vi "WSVCAP SHL Host TL RFFE Write - Multiple DUTs - Common Data.vi"(0 "Data Out":string, 11 "error in":errorcluster, 12 "FPGA":T1, 13 "DUT Mask (All)":bool[](array[boolean])=[TRUE, TRUE, TRUE, TRUE, TRUE, TRUE, TRUE, TRUE, TRUE, TRUE, TRUE, TRUE, TRUE, TRUE, TRUE, TRUE, TRUE, TRUE, TRUE, TRUE, TRUE, TRUE, TRUE, TRUE, TRUE, TRUE, TRUE, TRUE, TRUE, TRUE, TRUE, TRUE, TRUE, TRUE, TRUE, TRUE], 14 "Log (T)":bool=TRUE) -> (15 "error out":errorcluster)   [LabVIEW 2012]
uses:
  Type Defs/WSVCAP SHL I2C FPGA Enum.ctl
panel:
  out "Socket Mask":u64=1 format="%02x"
  out "RFFE Data Out [U8]":u8[][](array[numeric]) format="%02x"
  # "DUT 01"
  # "DUT 02"
  # "DUT 03"
  # "DUT 04"
  # "DUT 05"
  # "DUT 06"
  # "DUT 07"
  # "DUT 08"
  # "DUT 09"
  # "DUT 10"
  # "DUT 11"
  # "DUT 12"
  # "DUT 13"
  # "DUT 14"
  # "DUT 15"
  # "DUT 16"
  # "DUT 17"
  # "DUT 18"
  # "DUT 19"
  # "DUT 20"
  # "DUT 21"
  # "DUT 22"
  # "DUT 23"
  # "DUT 24"
  # "DUT 25"
  # "DUT 26"
  # "DUT 27"
  # "DUT 28"
  # "DUT 29"
  # "DUT 30"
  # "DUT 31"
  # "DUT 32"
  # "DUT 33"
  # "DUT 34"
  # "DUT 35"
  # "DUT 36"
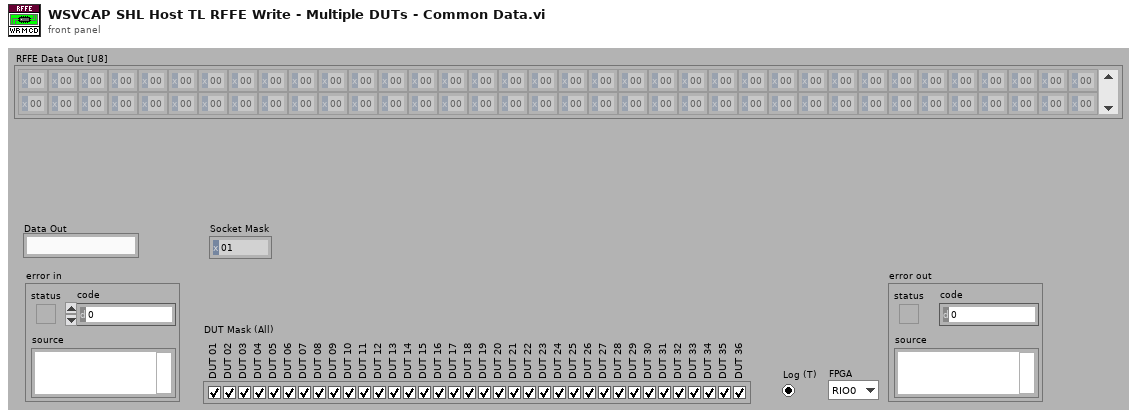
[diagram p1: front panel]
types:
  T1 = typedef "WSVCAP SHL I2C FPGA Enum.ctl" = enum16{"RIO0", "RIO1"}
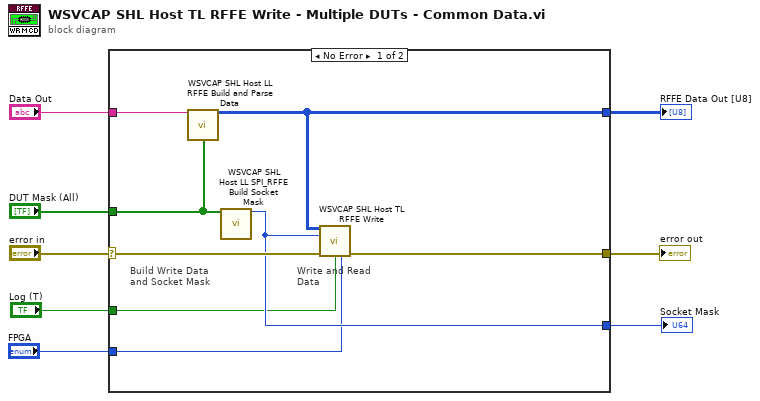
[diagram p0: block diagram]
diagram:
  n1 = case shown="No Error" "error in" {
    selector: "error in" -> [w15 _]
    tunnel: [w16 _] -> w8
    tunnel: "Data Out" -> [w14 _]
    tunnel: [w12 _] -> w5
    tunnel: [w11 _] -> w4
    tunnel: "DUT Mask (All)" -> [w13 _]
    tunnel: "Log (T)" -> [w10 _]
    tunnel: "FPGA" -> [w9 _]
    frame No Error {
      # "Write and Read\nData"
      # "Build Write Data and Socket Mask"
      n2 = call "WSVCAP SHL Host LL RFFE Build and Parse Data.vi"("Data Out"=w14, "DUT Mask (All)"=w13) -> ("RFFE Data Out [U8]"=w12:u8[][])  [unwired: 10 in, 3 out]
      n3 = call "WSVCAP SHL Host LL SPI_RFFE Build Socket Mask.vi"("DUT Mask"=w13) -> ("Socket Mask [U64]"=w11:u64)  [unwired: 14 in]
      n4 = call "WSVCAP SHL Host TL RFFE Write.vi"("RFFE Data Out"=w12, "Socket Mask"=w11, "error in"=w15, "Log (T)"=w10, "FPGA"=w9) -> ("error out"=w16:errorcluster)  [unwired: 10 in]
    }
    frame Error {
    }
  }
  "error out" <- w8
  "RFFE Data Out [U8]" <- w5
  "Socket Mask" <- w4
